vi "题目1.vi"() -> ()   [LabVIEW 2017]
panel:
  out "添加的数组":dbl[](array[numeric])
  out "元素 4":dbl
  out "元素 3":dbl
  out "元素 2":dbl
  out "元素":dbl
  out "数组":dbl[](array[numeric])
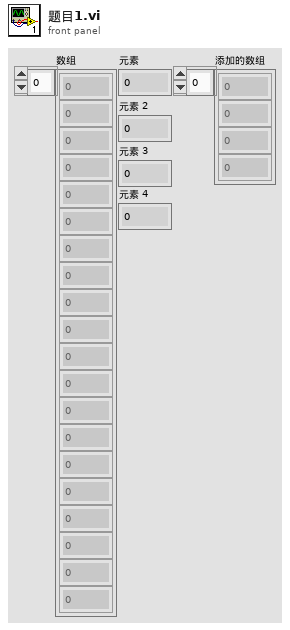
[diagram p1: front panel]
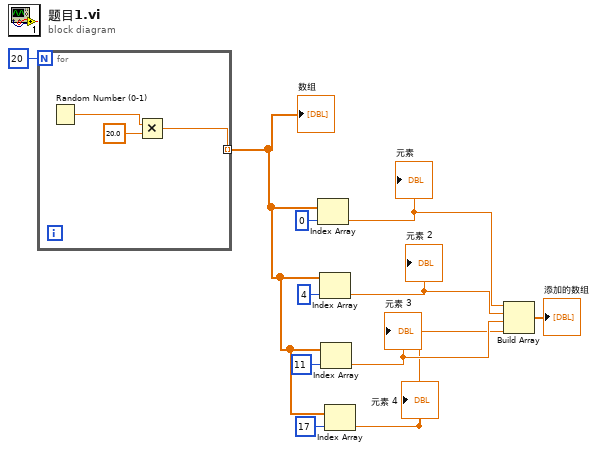
[diagram p0: block diagram]
diagram:
  n1 = for {
    N: 20 -> [_]
    tunnel: [w12] -> w9 mode=indexing
    n2 = Random Number (0-1)() -> (number: 0 to 1=w13:dbl)
    n3 = Multiply(x=w13, y=20.0) -> (x*y=w12:dbl)
  }
  "数组" <- w9
  n4 = Index Array(array=w9, index=0 ("索引")) -> (element=w5:dbl)
  "元素" <- w5
  n5 = Index Array(array=w9, index=4 ("索引")) -> (element=w4:dbl)
  "元素 2" <- w4
  n6 = Index Array(array=w9, index=11 ("索引")) -> (element=w3:dbl)
  "元素 3" <- w3
  n7 = Index Array(array=w9, index=17 ("索引")) -> (element=w2:dbl)
  "元素 4" <- w2
  n8 = Build Array(w5, w4, w3, w2) -> (→"添加的数组":dbl[])
